vi "Get target point on path.vi"(6 "Odometry":T1, 8 "Error Adapt? (F)":bool, 9 "index in":i32, 10 "Distance":dbl, 11 "Path in":T2[](array[typedef])) -> (1 "target index":i32, 2 "found?":bool, 3 "Path out":T2[](array[typedef]))   [LabVIEW 2019, in "Pure Pursuit.lvlib"]
uses:
  Pure Pursuit.lvlib
  Typedef/Path Point.ctl
  Odometry/Typedef/Odometry.ctl
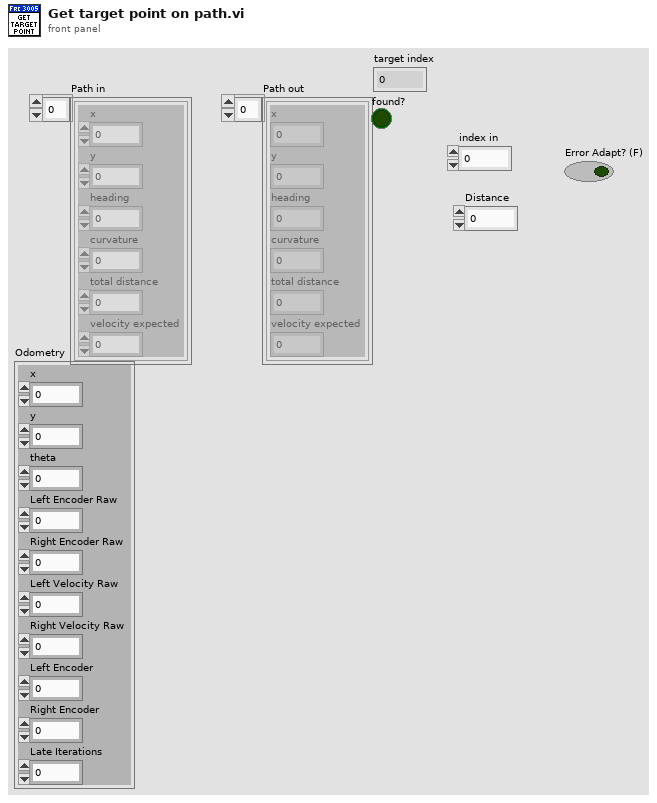
[diagram p1: front panel]
types:
  T1 = typedef "Odometry.ctl" = cluster{"x":dbl, "y":dbl, "theta":dbl, "Left Encoder Raw":i32, "Right Encoder Raw":i32, "Left Velocity Raw":i32, "Right Velocity Raw":i32, "Left Encoder":dbl, "Right Encoder":dbl, "Late Iterations":i16}
  T2 = typedef "Pure Pursuit.lvlib/Path Point.ctl" = cluster{"x":dbl, "y":dbl, "heading":dbl, "curvature":dbl, "total distance":dbl, "velocity expected":dbl}
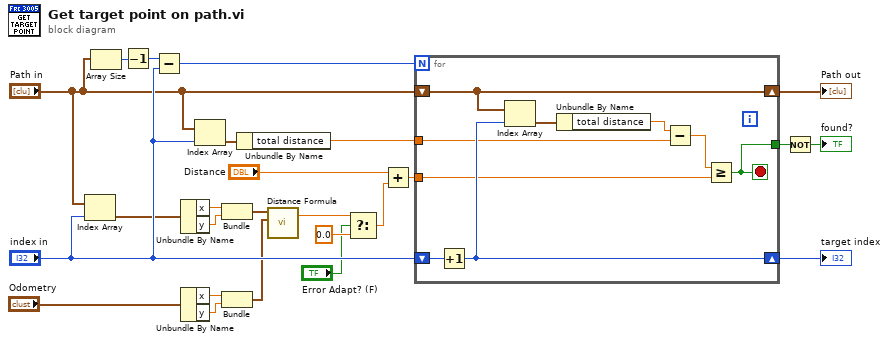
[diagram p0: block diagram]
diagram:
  n1 = Index Array(array="Path in", index="index in") -> (element=w9:T2)
  n2 = Array Size(array="Path in") -> (size(s)=w23:i32)
  n3 = Decrement(x=w23) -> (x-1=w22:i32)
  n4 = Subtract(x=w22, y="index in") -> (x-y=w24:i32)
  n5 = Unbundle By Name(w9) -> ("x"=w12:dbl, "y"=w11:dbl)
  n6 = Unbundle By Name("Odometry") -> ("x"=w7:dbl, "y"=w8:dbl)
  n7 = Index Array(array="Path in", index="index in") -> (element=w25:T2)
  n8 = Bundle("x"=w12, "y"=w11) -> (w10:cluster{"x":dbl, "y":dbl})  [unwired: 1 in]
  n9 = Bundle("x"=w7, "y"=w8) -> (w6:cluster{"x":dbl, "y":dbl})  [unwired: 1 in]
  n10 = Unbundle By Name(w25) -> ("total distance"=w20:dbl)
  n11 = call "Distance Formula.vi"("Point2"=w6, "Point1"=w10) -> ("Distance"=w2:dbl)  [unwired: 3 in]
  n12 = Select(t=w2, s="Error Adapt? (F)", f=0.0) -> (s? t:f=w1:dbl)
  n13 = Add(x="Distance", y=w1) -> (x+y=w15:dbl)
  n14 = for {
    N: w24 -> [_]
    shift-right: [w33] -> w21
    shift-left: "Path in" -> [w33]
    shift-right: [w32] -> w18
    shift-left: "index in" -> [w34]
    tunnel: w20 -> [w29]
    tunnel: w15 -> [w27]
    tunnel: [w26] -> w17
    stop <- w26 stop-if-true
    n15 = Increment(x=w34) -> (x+1=w32:i32)
    n16 = Index Array(array=w33, index=w32) -> (element=w31:T2)
    n17 = Unbundle By Name(w31) -> ("total distance"=w30:dbl)
    n18 = Subtract(x=w30, y=w29) -> (x-y=w28:dbl)
    n19 = Greater Or Equal?(x=w28, y=w27) -> (x >= y?=w26:bool)
  }
  "Path out" <- w21
  "target index" <- w18
  n20 = Not(x=w17) -> (.not. x?=→"found?":bool)
